vi "append horizontal lines to plot array.vi"(4 "BluePlotHandle":refnum<class "RocketPlotHandle.lvclass">, 6 "Plot ref":refnum<vi>, 7 "update plot":T1, 8 "error in (no error)":errorcluster, 9 "Newest Time to Plot (unix,ns)":u64, 10 "Oldest Time to Plot (unix,ns)":u64, 11 "top array":T5[](array[typedef])) -> (0 "error out":errorcluster, 1 "Numerics":dbl[](array[numeric]), 3 "Plot (LV epoch)":cluster{dbl[], "Data":dbl[]}[](array[cluster]), 5 "RightClickCache.slice":T4[](array[typedef]))   [LabVIEW 2021, in "RocketPlot.lvlib"]
uses:
  RocketPlot.lvlib
  TypeDefs/Plot top row.ctl
  Classes/RocketPlotHandle/RocketPlotHandle.lvclass
  TypeDefs/Slice average.ctl
  TypeDefs/update plot queue data.ctl
  TypeDefs/RightClickType.ctl
  <vilib>/Utility/miscctls.llb/LVPoint32TypeDef.ctl
  plot Unix to LV epoch.vi/3a8248cf-bec7-4c8d-a232-b35239452a92.vi
  plot Unix to LV epoch.vi/6d88088e-0f8c-482f-b724-f15eac533201.vi
  Decimate calc factors.vi
  Decimate data.vi/10c546bb-84c8-4f1e-93dc-e9aef4c9908a.vi
  Slice Average calc.vi
  Slice Average calc wrapper.vi/b0f39d84-27d9-4b84-b8c3-cf78f35fa78a.vi
  Slice Average calc wrapper.vi/b8f4d68e-665a-4d51-938f-4be5908799fb.vi
  Slice Average calc wrapper.vi/0a7e6c96-3213-4357-8ae2-7647ccf6d38e.vi
  Slice Average calc wrapper.vi/de1cbfd4-f4b0-4655-8da2-e779fdd6673d.vi
  <userlib>/bjustice/Ring Buffer for Time Series Data Strict Accessor/Unix time epoch/Unix_Epoch_in_Labview.vi
  <userlib>/bjustice/Ring Buffer for Time Series Data Strict Accessor/SubVIs/Search for time to keep.vi
  Slice Average calc.vi/aeb3b9b0-3d0b-48fb-8ca9-3c9e8c208765.vi
  Slice Average calc.vi/43998882-4a9d-44ca-a800-b6f182c48d79.vi
  <userlib>/bjustice/Ring Buffer for Time Series Data Strict Accessor/SubVIs/Search for oldest time to keep.vi
  <userlib>/bjustice/Ring Buffer for Time Series Data Strict Accessor/SubVIs/Search for newest time to keep.vi
  <vilib>/Analysis/baseanly.llb/Std Deviation and Variance.vi
  <vilib>/Analysis/8numeric.llb/Uneven Numeric Integration.vi
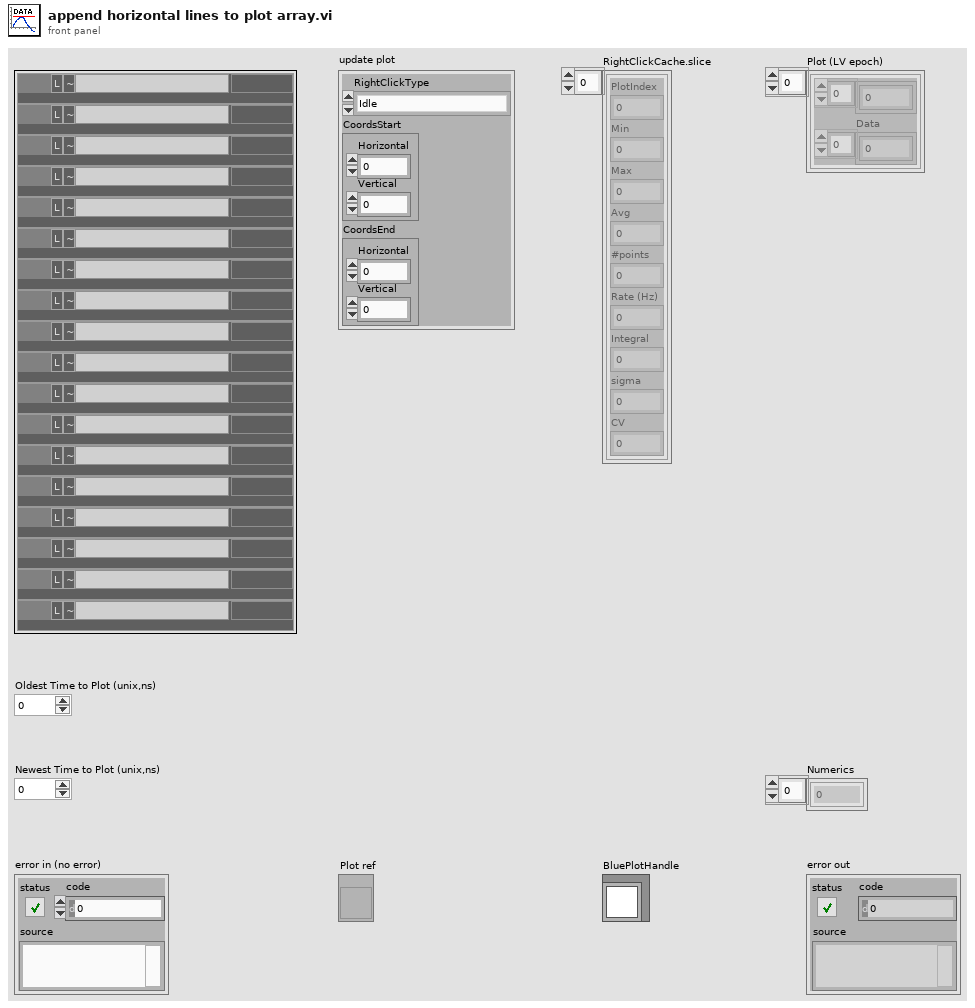
[diagram p1: front panel]
types:
  T1 = typedef "RocketPlot.lvlib/update plot queue data.ctl" = cluster{"RightClickType":T2, "CoordsStart":T3, "CoordsEnd":T3}
  T2 = typedef "RocketPlot.lvlib/RightClickType.ctl" = enum16{"Idle", "Delta", "SliceAvg", "Identify"}
  T3 = typedef "LVPoint32TypeDef.ctl" = cluster{"Horizontal":i32, "Vertical":i32}
  T4 = typedef "RocketPlot.lvlib/Slice average.ctl" = cluster{"PlotIndex":i32, "Min":dbl, "Max":dbl, "Avg":dbl, "#points":u32, "Rate (Hz)":dbl, "Integral":dbl, "sigma":dbl, "CV":dbl}
  T5 = typedef "RocketPlot.lvlib/Plot top row.ctl" = cluster{"PID":string, "index":i32, "PID color":u32, "right axis?":bool, "Flatline?":bool, "Numeric color":u32, "Data":string, "Flat":string}
  T6 = typedef "RocketPlot.lvlib/plot datapoint.ctl" = cluster{"Timestamps":u64[], "Data":dbl[]}
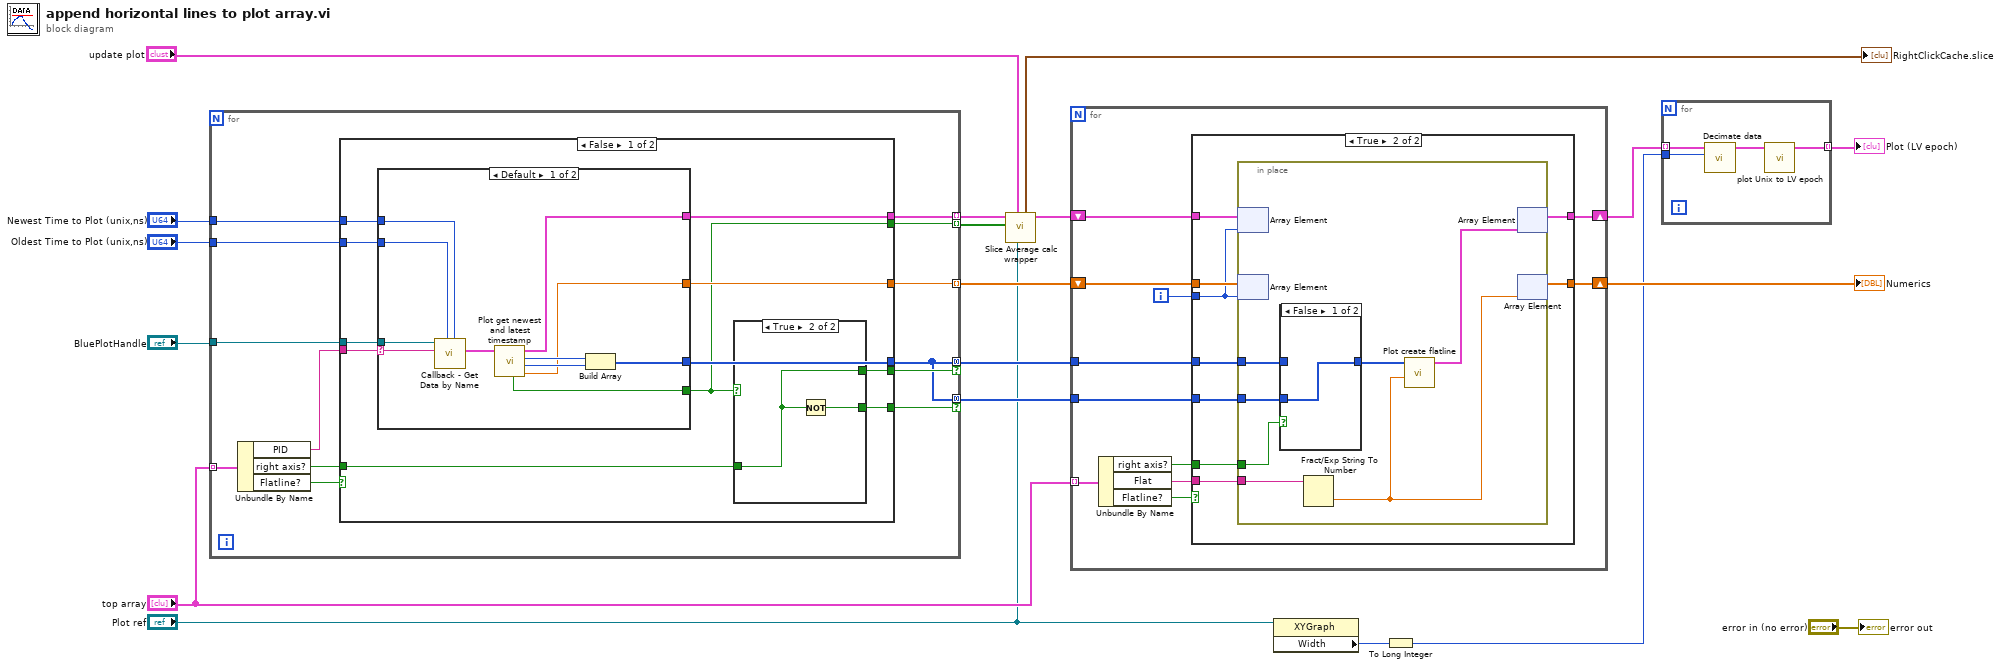
[diagram p0: block diagram]
diagram:
  n1 = for {
    tunnel: "top array" -> [w30] mode=indexing
    tunnel: [w32] -> w8 mode=indexing
    tunnel: [w31] -> w18 mode=indexing
    tunnel: [w25] -> w16 mode=concatenating if=w26
    tunnel: [w25] -> w15 mode=concatenating if=w24
    tunnel: "BluePlotHandle" -> [w23]
    tunnel: "Oldest Time to Plot (unix,ns)" -> [w22]
    tunnel: "Newest Time to Plot (unix,ns)" -> [w21]
    tunnel: [w20] -> w6 mode=indexing
    n2 = Unbundle By Name(w30) -> ("PID"=w29:string, "right axis?"=w27:bool, "Flatline?"=w28:bool)
    n3 = case shown="False" w28 {
      tunnel: [w43 _] -> w32
      tunnel: [w42 _] -> w31
      tunnel: w29 -> [w41 _]
      tunnel: [w40 _] -> w25
      tunnel: w27 -> [w39 _]
      tunnel: [w34 _] -> w26
      tunnel: [w38 _] -> w24
      tunnel: w23 -> [w37 _]
      tunnel: w22 -> [w36 _]
      tunnel: w21 -> [w35 _]
      tunnel: [w33 _] -> w20
      frame False {
        n4 = case shown="Default" w41 {
          selector: w41 -> [w45 _]
          tunnel: [w54 _] -> w43
          tunnel: [w50 _] -> w42
          tunnel: [w52 _] -> w40
          tunnel: w37 -> [w49 _]
          tunnel: w36 -> [w47 _]
          tunnel: w35 -> [w46 _]
          tunnel: [w44 _] -> w33
          frame Default {
            n5 = call-dynamic "Callback - Get Data by Name.vi"("Newest Time to Plot (unix,ns)"=w46, "Oldest Time to Plot (unix,ns)"=w47, "Name"=w45, "BluePlotHandle in"=w49) -> ("data history"=w48:T6)  [unwired: 5 in, 2 out]
            n6 = call "Plot get newest and latest timestamp.vi"("data history"=w48) -> ("newest data"=w50:dbl, "newest timestamp"=w51:u64, "oldest timestamp"=w53:u64, "data history"=w54:T6, "Exists?"=w44:bool)  [unwired: 6 in]
            n7 = Build Array(w53, w51) -> (w52:u64[])
          }
          frame "" {
          }
        }
        n8 = case shown="True" w33 {
          tunnel: w39 -> [_ w55]
          tunnel: [_ w56] -> w38
          tunnel: [_ w55] -> w34
          frame False {
          }
          frame True {
            n9 = Not(x=w55) -> (.not. x?=w56:bool)
          }
        }
      }
      frame True {
      }
    }
  }
  n10 = call "Slice Average calc wrapper.vi"("Plot ref"="Plot ref", "update plot"="update plot", "HasData?"=w6, "Plot (unix)"=w8) -> ("Plot (unix)"=w7:T6[], "RightClickCache.slice"=→"RightClickCache.slice":T4[])  [unwired: 6 in]
  n11 = for {
    tunnel: "top array" -> [w67] mode=indexing
    shift-right: [w63] -> w9
    shift-left: w7 -> [w65]
    shift-right: [w62] -> w17
    shift-left: w18 -> [w64]
    tunnel: w16 -> [w58]
    tunnel: w15 -> [w57]
    i -> [w59]
    n12 = Unbundle By Name(w67) -> ("right axis?"=w60:bool, "Flat"=w61:string, "Flatline?"=w66:bool)
    n13 = case shown="True" w66 {
      tunnel: w65 -> [w69 w78]
      tunnel: w64 -> [w68 w76]
      tunnel: [w69 w77] -> w63
      tunnel: [w68 w75] -> w62
      tunnel: w61 -> [_ w74]
      tunnel: w60 -> [_ w73]
      tunnel: w59 -> [_ w72]
      tunnel: w58 -> [_ w71]
      tunnel: w57 -> [_ w70]
      frame False {
      }
      frame True {
        n14 = in-place {
          in-place-border: w74 -> [w80]
          in-place-border: w73 -> [w84]
          in-place-border: w71 -> [w82]
          in-place-border: w70 -> [w81]
          n15 = in-place-array #1(w78, w72) -> ()  [unwired: 1 out]
          n16 = in-place-array #2(w76, w72) -> ()  [unwired: 1 out]
          n17 = case shown="False" w84 {
            tunnel: [w86 w87] -> w83
            tunnel: w82 -> [_ w87]
            tunnel: w81 -> [w86 _]
            frame False {
            }
            frame True {
            }
          }
          n18 = Fract/Exp String To Number(string=w80) -> (number=w79:dbl)  [unwired: 3 in, 1 out]
          n19 = call "Plot create flatline.vi"("value"=w79, "oldest,newest timestamp"=w83) -> ("data history"=w85:T6)  [unwired: 9 in]
          n20 = in-place-array #1(w85) -> (w77:T6[])  [unwired: 1 out]
          n21 = in-place-array #2(w79) -> (w75:dbl[])  [unwired: 1 out]
        }
      }
    }
  }
  "Numerics" <- w17
  n22 = property class="XYGraph"(reference="Plot ref") -> ("Width"=w5:u32)  [unwired: 1 in, 2 out]
  n23 = To Long Integer(number=w5) -> (32bit integer=w3:i32)
  n24 = for {
    tunnel: w9 -> [w88] mode=indexing
    tunnel: [w91] -> w13 mode=indexing
    tunnel: w3 -> [w89]
    n25 = call "Decimate data.vi"("Plot Area:Size:Width"=w89, "Plot (unix)"=w88) -> ("Plot (unix)"=w90:T6)  [unwired: 9 in]
    n26 = call "plot Unix to LV epoch.vi"("Plot (unix)"=w90) -> ("Plot (LV epoch)"=w91:cluster{dbl[], "Data":dbl[]})  [unwired: 10 in]
  }
  "Plot (LV epoch)" <- w13
  "error out" <- "error in (no error)"
